vi "CMN_SetUnscError.vi"(8 "error in (no error)":errorcluster, 10 "unsc error":errorcluster, 11 "Database RefNum in":T1) -> (0 "error out":errorcluster)   [LabVIEW 2016]
uses:
  DBSHAND/private/vis/DatabaseHand_RefNum.ctl
  DBSHAND/private/vis/DatabaseHand_Element_Set(error).vi
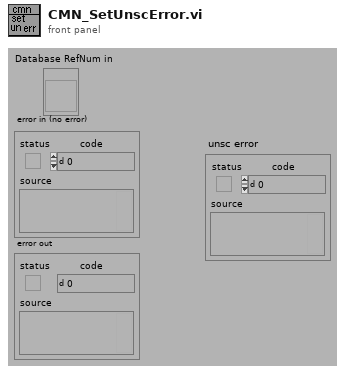
[diagram p1: front panel]
types:
  T1 = typedef "DatabaseHand_RefNum.ctl" = refnum<vi>
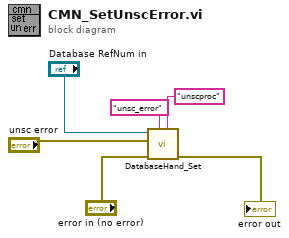
[diagram p0: block diagram]
diagram:
  n1 = call-poly "DatabaseHand_Set.vi"("group"="unscproc", "name"="unsc_error", "error in (no error)"="error in (no error)", "value"="unsc error", "Database RefNum in"="Database RefNum in") -> ("error out"=→"error out":errorcluster)  [unwired: 3 in, 3 out]
